vi "LcWebView_AlertDialog_Custom with a long content inside.vi"() -> ()   [LabVIEW 2018, in "LcWebView.lvclass"]
uses:
  LcWebView.lvclass
  webui/ctrls/AlertDialogWithImage.ctl
  C:/Program Files/National Instruments/LabVIEW 2020/user.lib/_LabVIEWCommon/LcWebView/LcWebView_class/data/Microsoft.Web.WebView2.WinForms.dll
panel:
  out "BrowserProcessId":u32
  in  "stop":bool
  out "Result":string
  out "Status Message":string
  in  "Web":refnum<k24>(container)
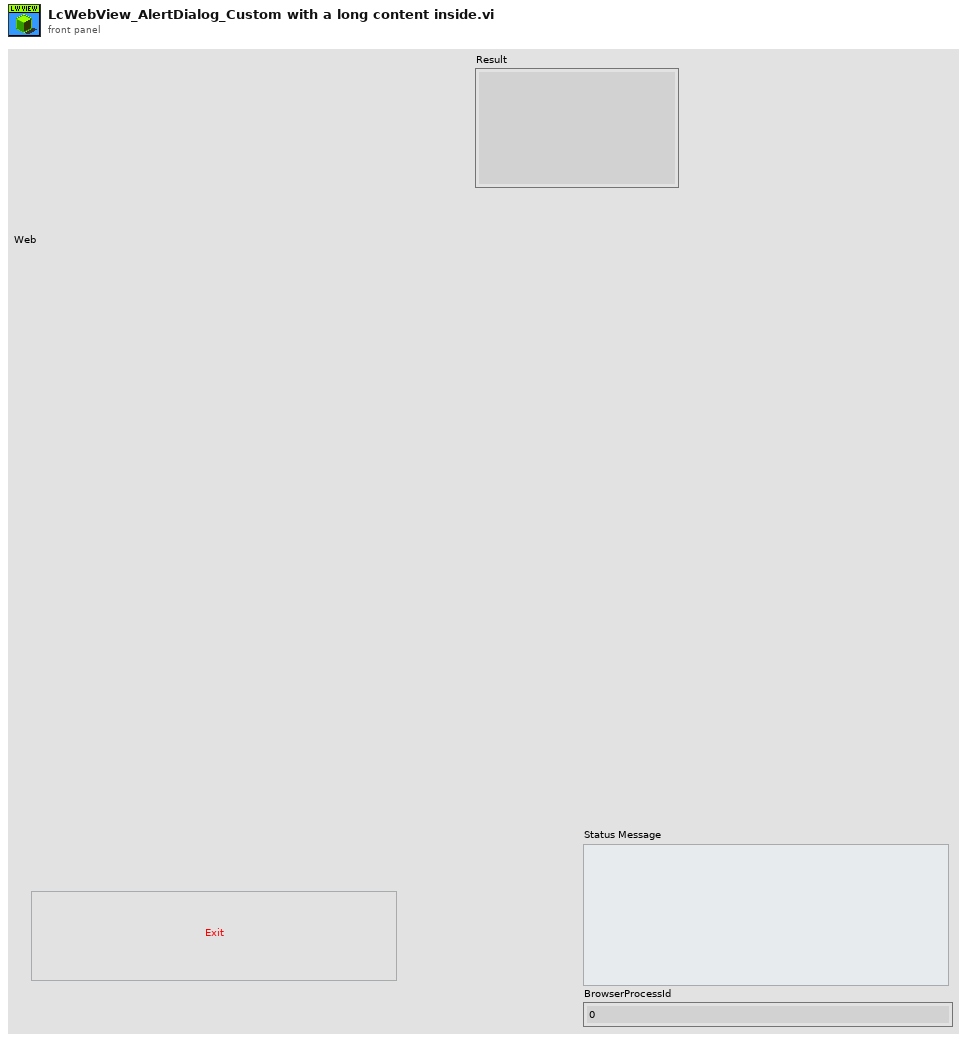
[diagram p1: front panel]
types:
  T1 = typedef "LcWebView.lvclass/AlertDialogWithImage.ctl" = cluster{"imageUrl":string, "imageAlt":string, "imageHeight":dbl}
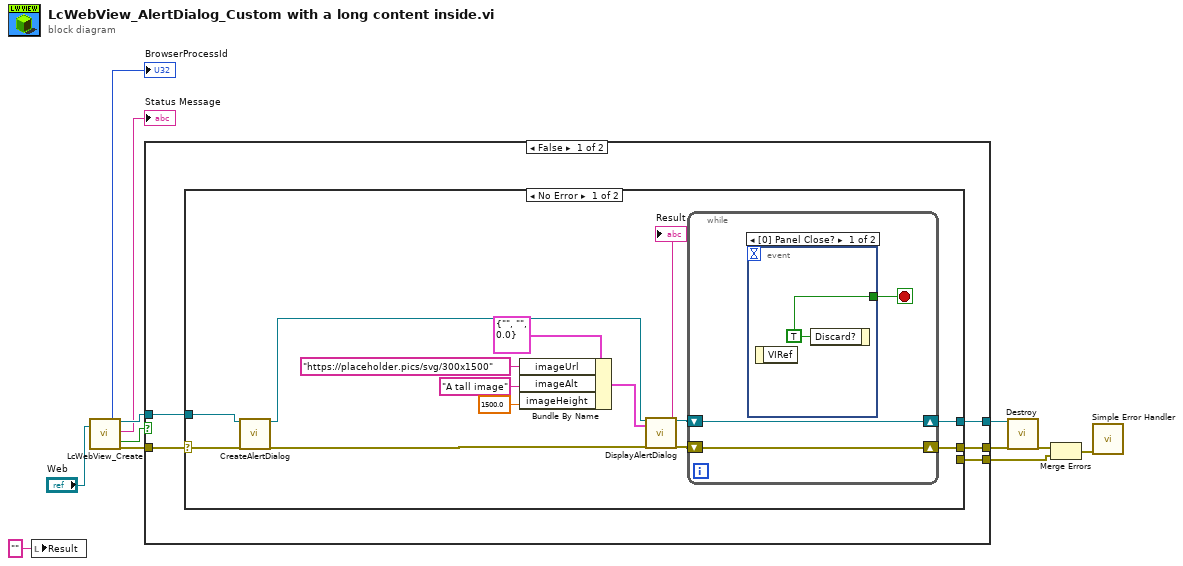
[diagram p0: block diagram]
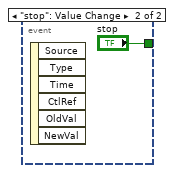
[diagram p2: hidden frame]
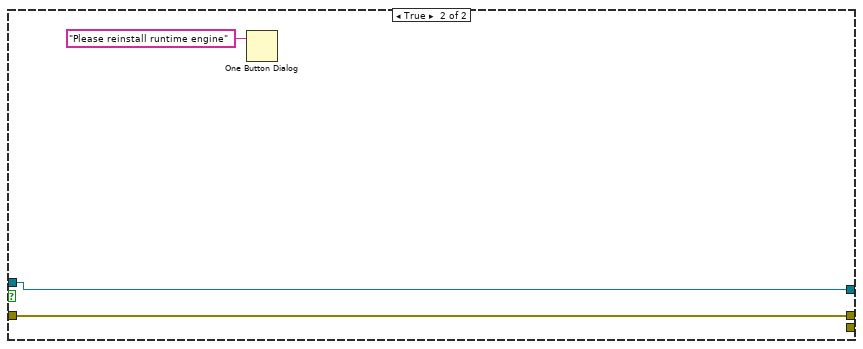
[diagram p4: hidden frame]
diagram:
  n1 = local write "Result"("" ("Result")) -> ()
  n2 = call "LcWebView_Create.vi"("Webview container"="Web") -> ("BrowserProcessId"=→"BrowserProcessId":u32, "reference out"=w11:refnum<class "LcWebView.lvclass">, "Status Message"=→"Status Message":string, "Reinstall Runtime"=w4:bool, "Error Out"=w10:errorcluster)  [unwired: 11 in, 3 out]
  n3 = case shown="False" w4 {
    tunnel: w11 -> [w17 w41]
    tunnel: w10 -> [w16 w40]
    tunnel: [w15 w41] -> w9
    tunnel: [w13 w40] -> w8
    tunnel: [w14 _] -> w5
    frame False {
      n4 = case shown="No Error" w16 {
        selector: w16 -> [w28 w37]
        tunnel: w17 -> [w29 w38]
        tunnel: [w30 w38] -> w15
        tunnel: [w31 _] -> w13
        tunnel: [_ w37] -> w14
        frame No Error {
          n5 = call-dynamic "CreateAlertDialog.vi"("reference in"=w29, "Error In"=w28) -> ("reference out"=w27:refnum<class "LcWebView.lvclass">, "Error Out"=w26:errorcluster)  [unwired: 16 in]
          n6 = Bundle By Name(cluster=T1 {"imageUrl"="", "imageAlt"="", "imageHeight"=0.0}, "imageUrl"="https://placeholder.pics/svg/300x1500", "imageAlt"="A tall image", "imageHeight"=1500.0) -> (w23:T1)
          n7 = call-dynamic "DisplayAlertDialog.vi"("reference in"=w27, "Message"=w23, "Error In"=w26) -> ("reference out"=w25:refnum<class "LcWebView.lvclass">, "Result"=→"Result":string, "Error Out"=w24:errorcluster)  [unwired: 14 in]
          n8 = while {
            shift-right: [w34] -> w30
            shift-left: w25 -> [w34]
            shift-right: [w33] -> w31
            shift-left: w24 -> [w33]
            stop <- w32 stop-if-true
            n9 = event shown="[0] Panel Close?" {
              selector: _ -> [_ _]
              dyn-events: _ -> [_ _]
              timeout: _ -> [_ _]
              tunnel: [w35 "stop"] -> w32
              event Panel Close? {
                w35 = TRUE ("Discard?")
                n10 = event-data() -> ()  [unwired: 1 in, 1 out]
                n11 = event-data("Discard?"=w35) -> ()  [unwired: 1 in, 1 out]
              }
              event "stop": Value Change {
                n12 = event-data() -> ()  [unwired: 1 in, 6 out]
              }
            }
          }
        }
        frame Error {
        }
      }
    }
    frame True {
      n13 = One Button Dialog(message="Please reinstall runtime engine") -> ()  [unwired: 1 in, 1 out]
    }
  }
  n14 = call-dynamic "Destroy.vi"("reference in"=w9, "Error In"=w8) -> ("Error Out"=w7:errorcluster)  [unwired: 16 in, 1 out]
  n15 = Merge Errors(w7, w5) -> (w2:errorcluster)
  n16 = call <vilib>:"Simple Error Handler.vi"("error in (no error)"=w2) -> ()  [unwired: 4 in, 5 out]
